vi "FestoCPX.Station.TowerHorn.Set.vi"(8 "error in":errorcluster, 10 "Horn (F)":bool, 11 "Period [s] (0)":dbl) -> (0 "error out":errorcluster)   [LabVIEW 2016]
uses:
  FestoCPX.DO.Signal.ctl
  FestoCPX.Station.TowerHorn.Fglb.Action.ctl
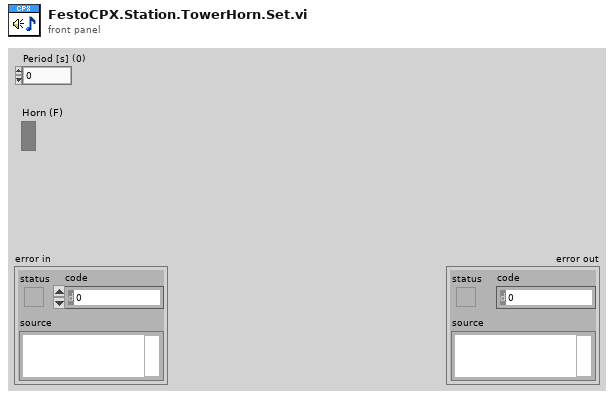
[diagram p1: front panel]
types:
  T1 = typedef "FestoCPX.DO.Signal.ctl" = enum16{"Safety Reset", "Air Main Valve", "Door Lock", "Button LED Start", "Button LED Stop", "Button LED Control", "Traffic LED Red", "Traffic LED Orange", "Traffic LED Green", "Horn", "Laser Interlock", "Laser Trigger", "Laser Fume Extractor", "Product Suction Gripper Slot 1 A", "Product Suction Gripper Slot 1 B", "Product Suction Gripper Slot 2 A", "Product Suction Gripper Slot 2 B", "Product Suction Gripper Slot 3 A", "Product Suction Gripper Slot 3 B", "Product Suction Gripper Slot 4 A", "Product Suction Gripper Slot 4 B", "Product Suction Gripper Final A", "Product Suction Gripper Final B", "Lamp", "Q1 Product Move Work", "Q1 Product Move Home", "Q2 Table Turn Work", "Q2 Table Turn Home", "Q3 Product Lift A", "Q3 Product Lift B", "Q4 Product Arm OK", "Q4 Product Arm NOK", "Q5 Product Arm Work", "Q6 Product BlowOut A", "Q6 Product BlowOut B"}
  T2 = typedef "FestoCPX.Station.TowerHorn.Fglb.Action.ctl" = enum16{"init", "set", "get"}
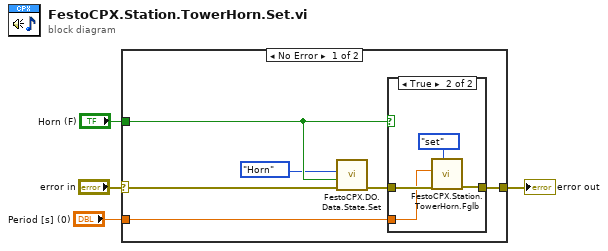
[diagram p0: block diagram]
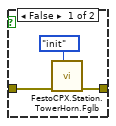
[diagram p2: hidden frame]
diagram:
  n1 = case shown="No Error" "error in" {
    selector: "error in" -> [w10 w18]
    tunnel: [w8 w18] -> w4
    tunnel: "Period [s] (0)" -> [w7 _]
    tunnel: "Horn (F)" -> [w6 _]
    frame No Error {
      n2 = call "FestoCPX.DO.Data.State.Set.vi"("error in (no error)"=w10, "State"=w6, "CPX.DO"=FestoCPX.DO.Signal."Horn") -> ("error out"=w9:errorcluster)  [unwired: 8 in]
      n3 = case shown="True" w6 {
        tunnel: w9 -> [w12 w16]
        tunnel: [w11 w15] -> w8
        tunnel: w7 -> [_ w14]
        frame False {
          n4 = call "FestoCPX.Station.TowerHorn.Fglb.vi"("Action (get)"=FestoCPX.Station.TowerHorn.Fglb.Action."init", "error in"=w12) -> ("error out"=w11:errorcluster)  [unwired: 8 in, 1 out]
        }
        frame True {
          n5 = call "FestoCPX.Station.TowerHorn.Fglb.vi"("Action (get)"=FestoCPX.Station.TowerHorn.Fglb.Action."set", "error in"=w16, "Period [s]"=w14) -> ("error out"=w15:errorcluster)  [unwired: 7 in, 1 out]
        }
      }
    }
    frame Error {
    }
  }
  "error out" <- w4
